vi "Read Return Address.vi"(8 "error in (no error)":errorcluster, 11 "Self Addressed Task in":refnum<class "Self Addressed Task.lvclass">) -> (0 "error out":errorcluster, 2 "Return Address":T1, 3 "Self Addressed Task out":refnum<class "Self Addressed Task.lvclass">)   [LabVIEW 2024, in "Self Addressed Task.lvclass"]
uses:
  Self Addressed Task.lvclass
  Type Def/Return Address.ctl
  Task Ancestor/Task Ancestor.lvclass
  Self Addressed Task.lvclass/Self Addressed Task.ctl
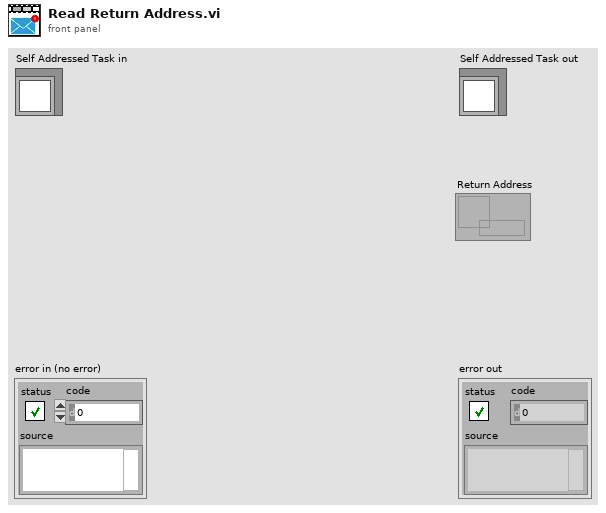
[diagram p1: front panel]
types:
  T1 = typedef "Return Address.ctl" = refnum<queue>
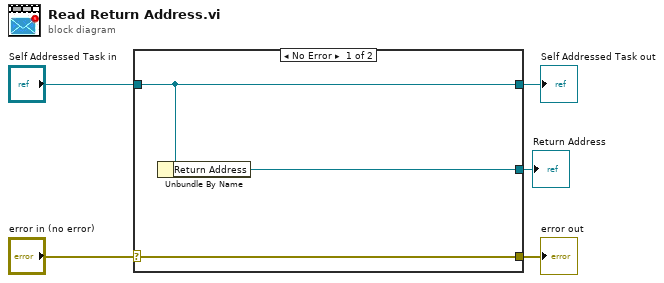
[diagram p0: block diagram]
diagram:
  n1 = case shown="No Error" "error in (no error)" {
    selector: "error in (no error)" -> [w8 w9]
    tunnel: [w8 w9] -> w4
    tunnel: [w7 w10] -> w2
    tunnel: "Self Addressed Task in" -> [w7 w10]
    tunnel: [w6 _] -> w1
    frame No Error {
      n2 = Unbundle By Name(w7) -> ("Return Address"=w6:T1)
    }
    frame Error {
    }
  }
  "error out" <- w4
  "Self Addressed Task out" <- w2
  "Return Address" <- w1
